vi "ShutOff_v00.vi"(2 "Debug Mode":bool, 3 "Elapsed Time(s)":dbl, 4 "State":enum16{"Edit", "Start", "Run", "End", "Idle"}(ring), 5 "Argument List In":string[](array[string])) -> (0 "Status Out":string, 1 "Argument List Out":string[](array[string]))   [LabVIEW 2011]
panel:
  out "total time":dbl
  out "is OK?":bool
  in  "Cancel":bool
  in  "OK":bool
  out "tTotal(s) 2":dbl
  # "Shuts off sources"
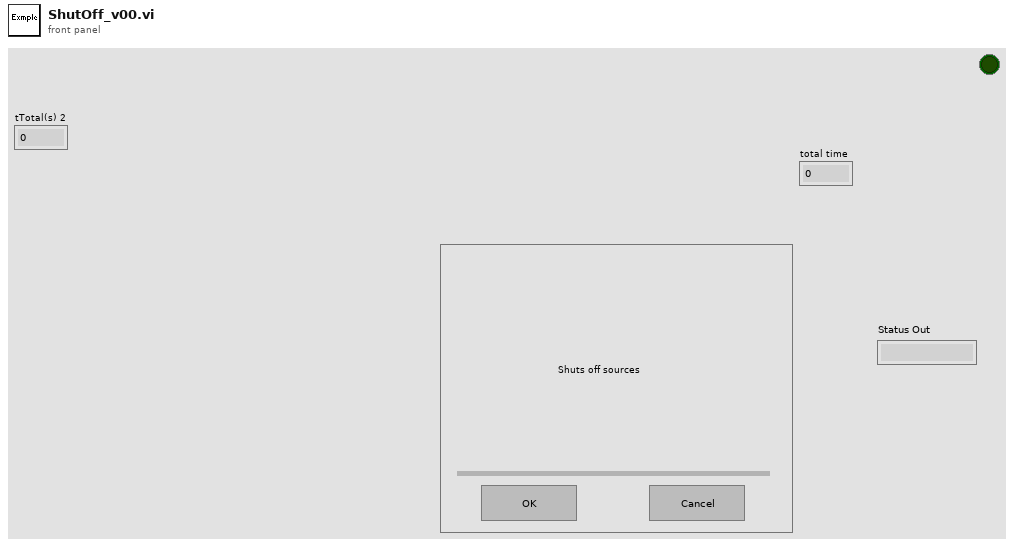
[diagram p1: front panel]
types:
  T1 = enum16{"Discrete", "Continuous", "Instantaneous", "Finite"}
  T2 = enum32{"Invalid", "Default", "Floating", "Floating/Auto-Hide", "Modal"}
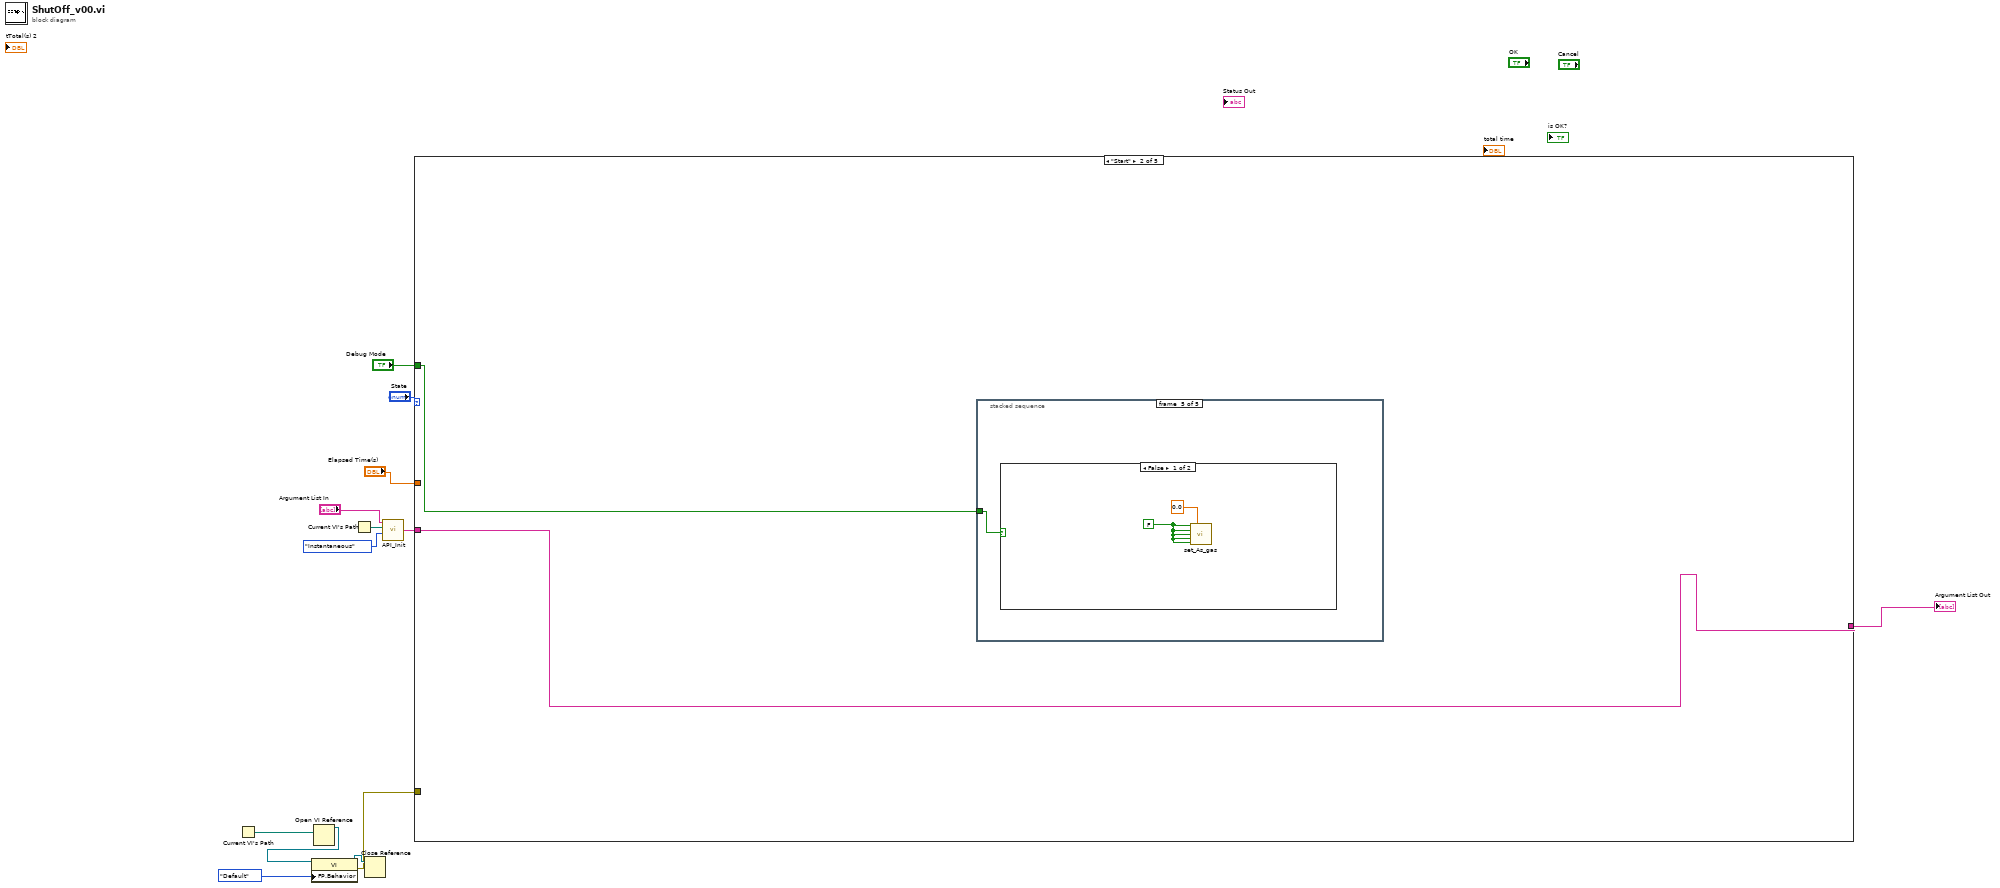
[diagram p0: block diagram]
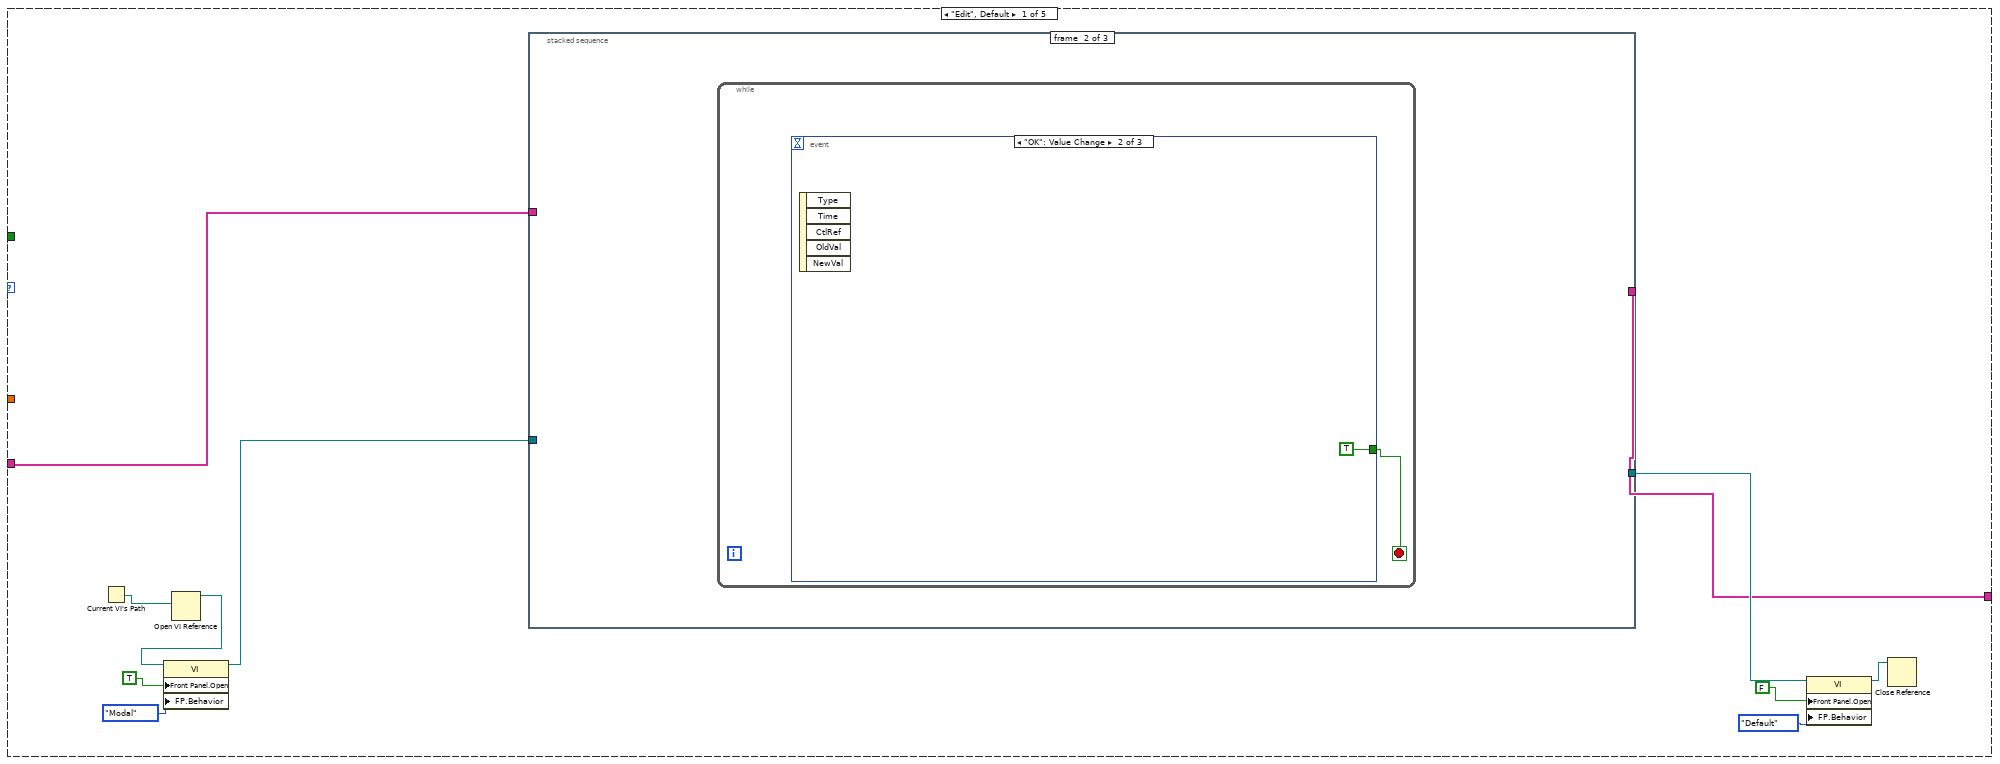
[diagram p2: hidden frame]
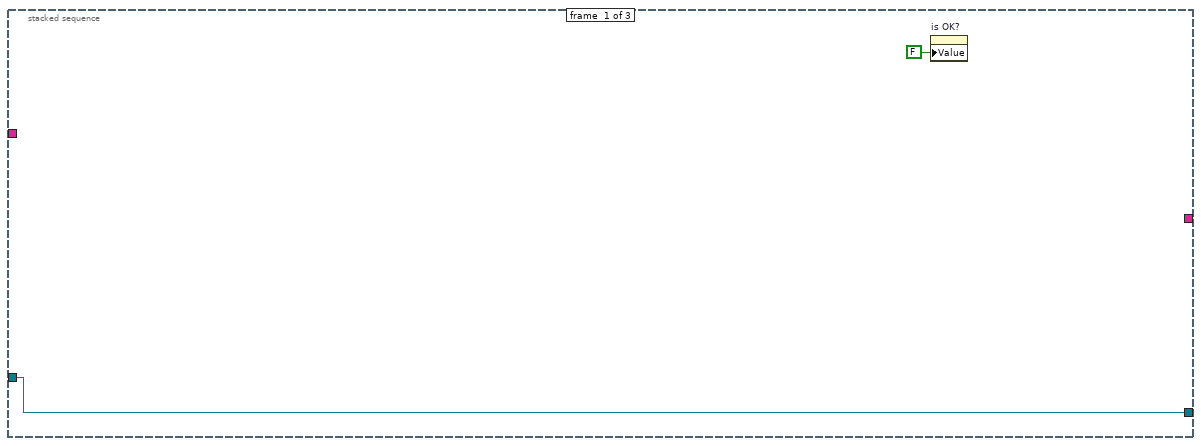
[diagram p3: hidden frame]
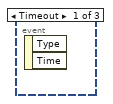
[diagram p4: hidden frame]
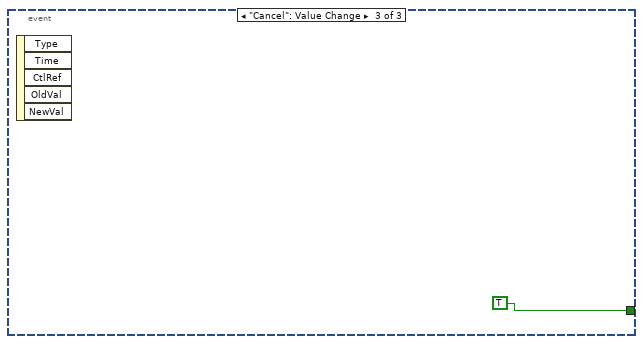
[diagram p5: hidden frame]
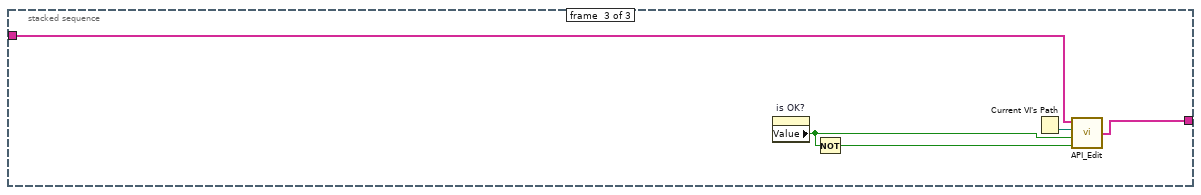
[diagram p6: hidden frame]
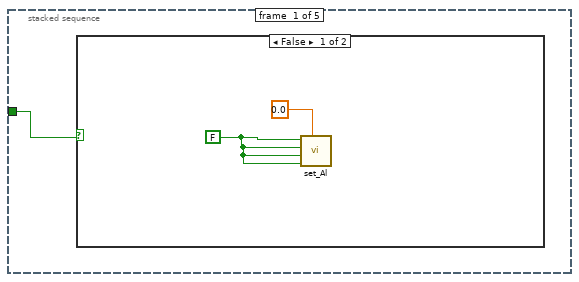
[diagram p7: hidden frame]
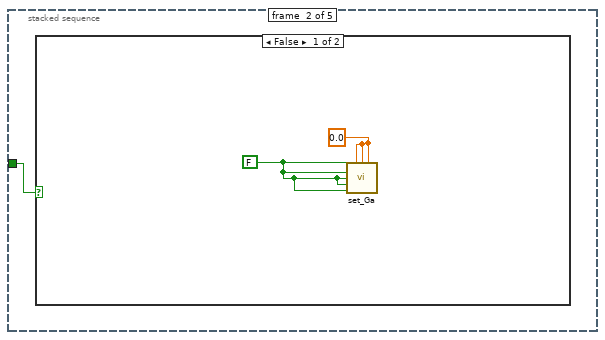
[diagram p9: hidden frame]
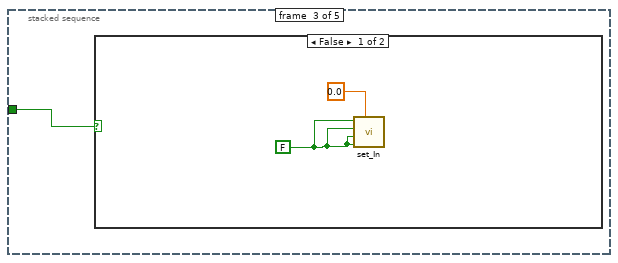
[diagram p11: hidden frame]
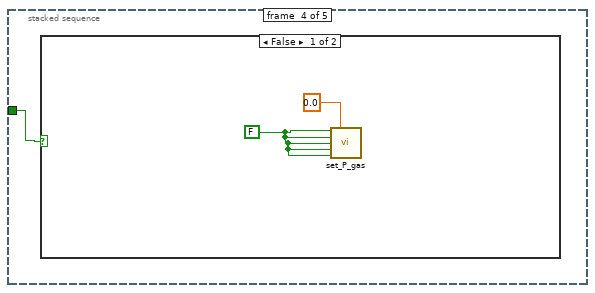
[diagram p13: hidden frame]
diagram:
  n1 = Current VI's Path() -> (path=w9:path)
  n2 = Open VI Reference(vi path=w9) -> (vi reference=w8:refnum<vi>)  [unwired: 1 in, 5 out]
  n3 = property class="VI"(reference=w8, "FP.Behavior"=T2."Default" ("Front Panel Window:Behavior")) -> (reference out=w6:refnum<vi>, error out=w5:errorcluster)  [unwired: 1 in]
  n4 = Current VI's Path() -> (path=w4:path)
  n5 = Close Reference(reference=w6) -> ()  [unwired: 1 in, 1 out]
  n6 = call "API_Init.vi"("API Mode"=T1."Instantaneous", "VI Path"=w4, "Argument List In"="Argument List In") -> ("Argument List Out"=w1:string[])  [unwired: 1 in]
  n7 = case shown="\"Start\"" "State" {
    tunnel: "Debug Mode" -> [_ w35 _ _ _]
    tunnel: "Elapsed Time(s)" -> [_ _ _ _ _]
    tunnel: w1 -> [w15 w36 w52 w53 w54]
    tunnel: [w14 w36 w52 w53 w54] -> w10
    tunnel: w5 -> [_ _ _ _ _]
    frame "Edit", Default {
      n8 = Current VI's Path() -> (path=w20:path)
      n9 = Open VI Reference(vi path=w20) -> (vi reference=w19:refnum<vi>)  [unwired: 1 in, 5 out]
      n10 = property class="VI"(reference=w19, "Front Panel.Open"=TRUE ("Front Panel Window:Open"), "FP.Behavior"=T2."Modal" ("Front Panel Window:Behavior")) -> (reference out=w18:refnum<vi>)  [unwired: 1 in, 1 out]
      n11 = stacked-sequence {
        tunnel: w15 -> [_ _ w30]
        tunnel: w18 -> [w26 _ _]
        tunnel: [w26 _ _] -> w22
        tunnel: [_ _ w32] -> w14
        frame #0 {
          n12 = property on="is OK?" class="Bool (strict)"("Value"=FALSE ("is OK?")) -> ()  [unwired: 2 in, 2 out]
        }
        frame #1 {
          n13 = while {
            stop <- w27 stop-if-true
            n14 = event shown="[1] \"OK\": Value Change" {
              selector: _ -> [_ _ _]
              dyn-events: _ -> [_ _ _]
              timeout: _ -> [_ _ _]
              tunnel: [_ TRUE TRUE] -> w27
              event Timeout {
                n15 = event-data() -> ()  [unwired: 1 in, 2 out]
              }
              event "OK": Value Change {
                n16 = event-data() -> ()  [unwired: 1 in, 5 out]
              }
              event "Cancel": Value Change {
                n17 = event-data() -> ()  [unwired: 1 in, 5 out]
              }
            }
          }
        }
        frame #2 {
          n18 = property on="is OK?" class="Bool (strict)"() -> ("Value"=w31:bool)  [unwired: 2 in, 2 out]
          n19 = Not(x=w31) -> (.not. x?=w34:bool)
          n20 = Current VI's Path() -> (path=w33:path)
          n21 = call "API_Edit.vi"("Cancel"=w34, "OK"=w31, "VI Path"=w33, "Argument List In"=w30) -> ("Argument List Out"=w32:string[])
        }
      }
      n22 = property class="VI"(reference=w22, "Front Panel.Open"=FALSE ("Front Panel Window:Open"), "FP.Behavior"=T2."Default" ("Front Panel Window:Behavior")) -> (reference out=w23:refnum<vi>)  [unwired: 1 in, 1 out]
      n23 = Close Reference(reference=w23) -> ()  [unwired: 1 in, 1 out]
    }
    frame "Start" {
      n24 = stacked-sequence {
        tunnel: w35 -> [w37 w40 w43 w46 w49]
        frame #0 {
          n25 = case shown="False" w37 {
            frame False {
              w39 = FALSE ("Al Active")
              n26 = call "set_Al.vi"("Aluminum Flow"=0.0, "Al Remote"=w39, "Al Run"=w39, "Al Bubbler"=w39, "Al Active"=w39) -> ()  [unwired: 5 out]
            }
            frame True {
            }
          }
        }
        frame #1 {
          n27 = case shown="False" w40 {
            frame False {
              w42 = FALSE ("Ga Active")
              w41 = 0.0 ("Ga Flow 1")
              n28 = call "set_Ga.vi"("Ga Active"=w42, "Ga Flow 3"=w41, "Ga Flow 2"=w41, "Ga Flow 1"=w41, "Ga Bubbler"=w42, "Ga H2 Dilute"=w42, "Ga Run"=w42, "Ga Remote"=w42) -> ()  [unwired: 8 out]
            }
            frame True {
            }
          }
        }
        frame #2 {
          n29 = case shown="False" w43 {
            frame False {
              w45 = FALSE ("In Remote")
              n30 = call "set_In.vi"("Indium Flow"=0.0, "In Remote"=w45, "In Run"=w45, "In Bubbler"=w45, "In Active"=w45) -> ()  [unwired: 5 out]
            }
            frame True {
            }
          }
        }
        frame #3 {
          n31 = case shown="False" w46 {
            frame False {
              w47 = FALSE ("P_Gas Active")
              n32 = call "set_P_gas.vi"("P_Gas Active"=w47, "P_Gas Flow"=0.0, "P_Gas In"=w47, "P_Gas H2 In"=w47, "P_Gas Run"=w47, "P_Gas Remote"=w47) -> ()  [unwired: 10 out]
            }
            frame True {
            }
          }
        }
        frame #4 {
          n33 = case shown="False" w49 {
            frame False {
              w50 = FALSE ("As_Gas Active")
              n34 = call "set_As_gas.vi"("As_Gas Active"=w50, "As_Gas Flow"=0.0, "As_Gas In"=w50, "As_Gas H2"=w50, "As_Gas Run"=w50, "As_Gas Remote"=w50) -> ()  [unwired: 10 in]
            }
            frame True {
            }
          }
        }
      }
    }
    frame "Run" {
    }
    frame "End" {
    }
    frame "Idle" {
    }
  }
  "Argument List Out" <- w10
